vi "Part_Image_Skewing2.vi"(4 "[IN] Cols":i32, 5 "[IN] Part shift":i32, 6 "[IN] tan(theta)":dbl, 7 "[IN] Source Image U16":u16[][](array[numeric]), 9 "[IN] Cols Initial":i32, 10 "[IN] Rows":i32, 11 "[IN] Rows Part":i32) -> (2 "[OUT] Pixel part":u16[][](array[numeric]))   [LabVIEW 2020]
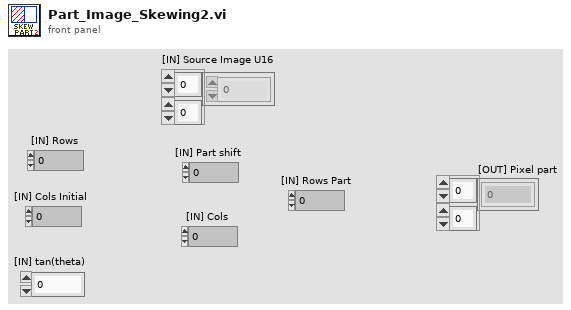
[diagram p1: front panel]
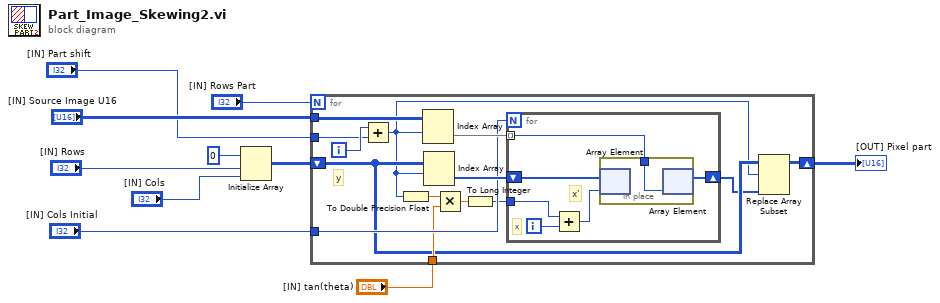
[diagram p0: block diagram]
diagram:
  n1 = Initialize Array(u16 0, "[IN] Rows", "[IN] Cols") -> (w10:u16[][])
  n2 = for {
    N: "[IN] Rows Part" -> [_]
    shift-right: [w15] -> w1
    shift-left: w10 -> [w16]
    tunnel: "[IN] Source Image U16" -> [w23]
    tunnel: "[IN] Cols Initial" -> [w21]
    tunnel: "[IN] tan(theta)" -> [w19]
    tunnel: "[IN] Part shift" -> [w12]
    i -> [w13]
    # "y"
    n3 = Add(x=w13, y=w12) -> (x+y=w11:i32)
    n4 = To Double Precision Float(number=w11) -> (double precision float=w20:dbl)
    n5 = Index Array(array=w23, index (row)=w11) -> (element=w22:u16[])  [unwired: 1 in]
    n6 = Index Array(array=w16, index (row)=w11) -> (element=w24:u16[])  [unwired: 1 in]
    n7 = Multiply(x=w20, y=w19) -> (x*y=w18:dbl)
    n8 = To Long Integer(number=w18) -> (32bit integer=w17:i32)
    n9 = for {
      N: w21 -> [_]
      shift-right: [w26] -> w14
      shift-left: w24 -> [w28]
      tunnel: w22 -> [w25] mode=indexing
      tunnel: w17 -> [w29]
      i -> [w30]
      # "x'"
      # "x"
      n10 = Add(x=w29, y=w30) -> (x+y=w27:i32)
      n11 = in-place {
        in-place-border: w25 -> [w31]
        n12 = in-place-array #1(w28, w27) -> ()  [unwired: 1 out]
        n13 = in-place-array #1(w31) -> (w26:u16[])  [unwired: 1 out]
      }
    }
    n14 = Replace Array Subset(array=w16, new element=w14, index (row)=w11) -> (w15:u16[][])  [unwired: 1 in]
  }
  "[OUT] Pixel part" <- w1
